vi "RegisterWindow.vi"() -> ()   [LabVIEW 2013]
panel:
  out "子字符串":string
  out "LicCode":string
  out "机器码":string
  out "Tip":string
  in  "注册码":string
  out "连接的字符串":string
  in  "退出":bool
  in  "注册":bool
  in  "簇":T1
  out "字符串":string
  out "鉴权通过":bool
  out "参数配置":bool
  out "参数生成":bool
  out "强制操作":bool
  out "数据保存":bool
  out "Times":dbl
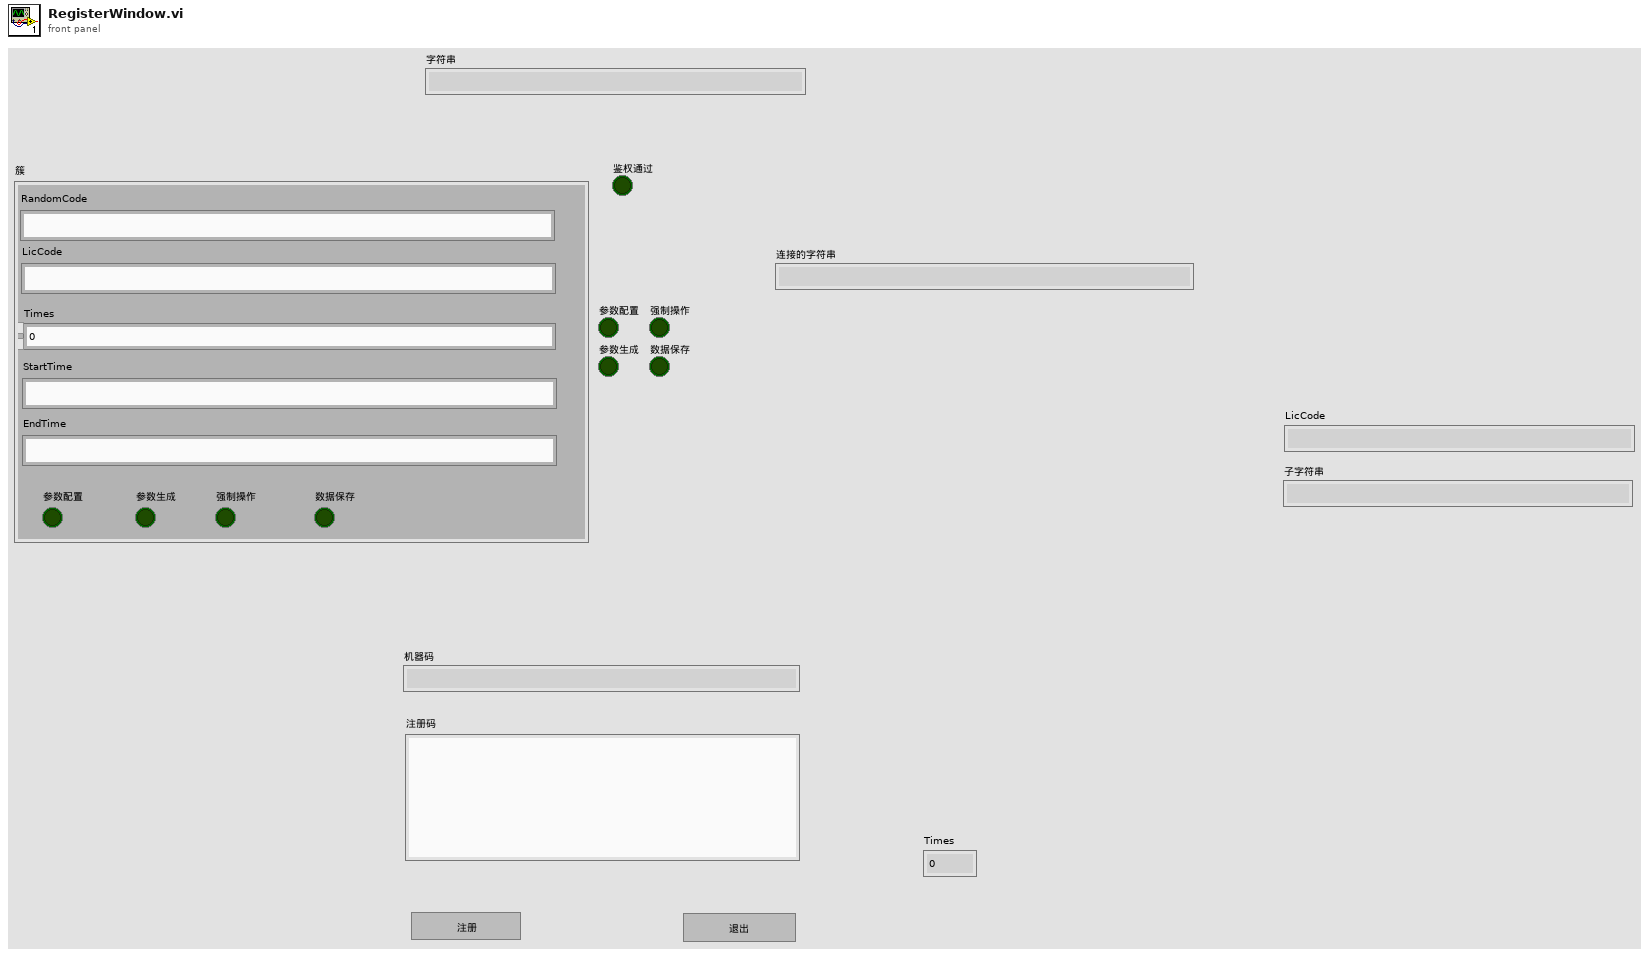
[diagram p1: front panel]
types:
  T1 = cluster{"RandomCode":string, "LicCode":string, "Times":dbl, "StartTime":string, "EndTime":string, "参数配置":bool, "参数生成":bool, "强制操作":bool, "数据保存":bool}
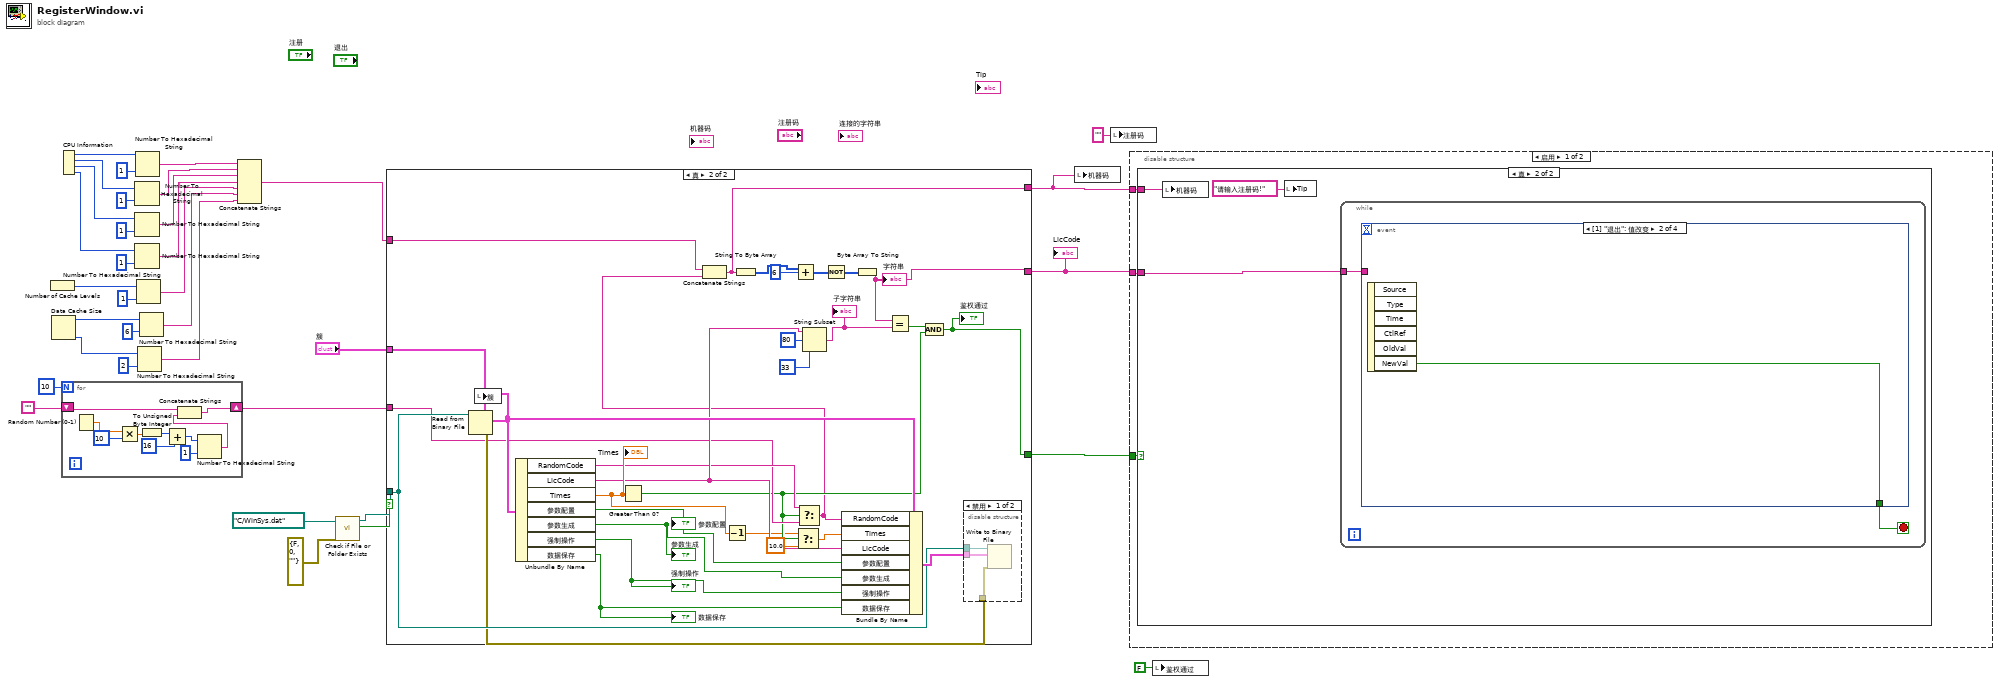
[diagram p0: block diagram]
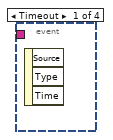
[diagram p3: hidden frame]
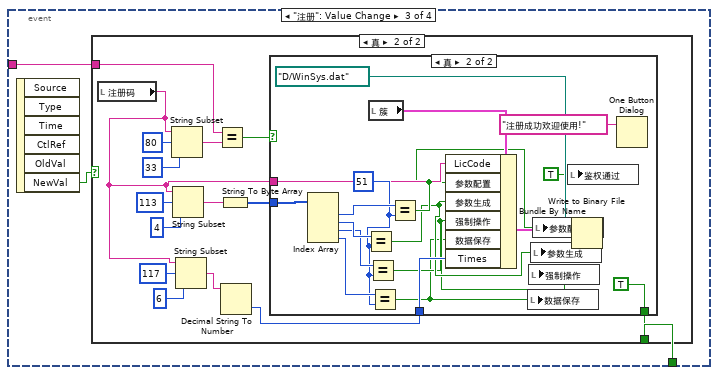
[diagram p4: hidden frame]
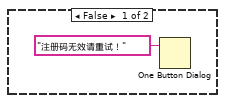
[diagram p6: hidden frame]
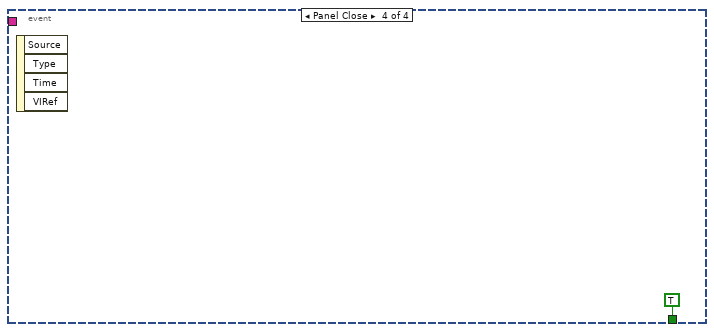
[diagram p7: hidden frame]
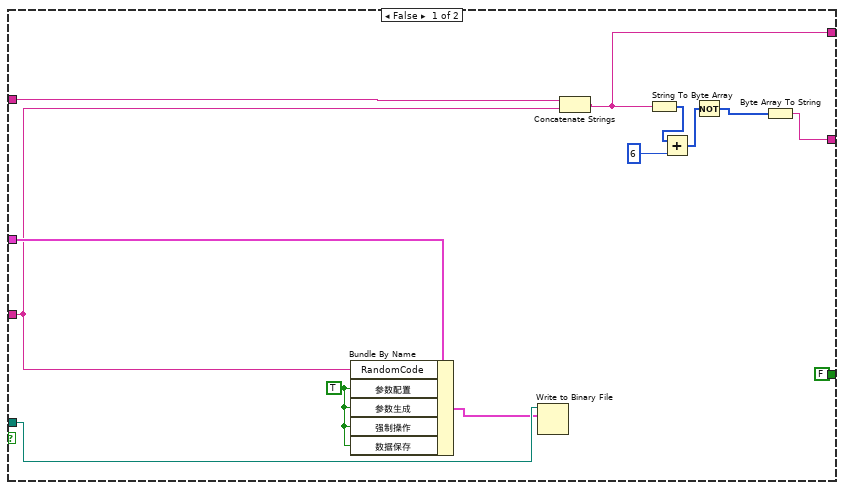
[diagram p9: hidden frame]
diagram:
  n1 = Number of Cache Levels() -> (w20:i32)
  n2 = Data Cache Size() -> (4:w21:i32, 7:w23:i32)  [unwired: 1 in]
  n3 = CPU Information() -> (4:w11:i32, 5:w15:i32, 6:w16:i32, 7:w17:i32)
  n4 = for {
    N: 10 -> [_]
    shift-right: [w37] -> w1
    shift-left: "" -> [w38]
    n5 = Random Number (0-1)() -> (number: 0 to 1=w45:dbl)
    n6 = Multiply(x=w45, y=u8 10) -> (x*y=w43:dbl)
    n7 = To Unsigned Byte Integer(number=w43) -> (unsigned 8bit integer=w41:u8)
    n8 = Add(x=w41, y=u8 16) -> (x+y=w39:u8)
    n9 = Number To Hexadecimal String(1:i16 1 ("宽度(-)"), 2:w39) -> (0:w36:string)
    n10 = Concatenate Strings(w38, w36) -> (w37:string)
  }
  n11 = Number To Hexadecimal String(1:i16 1 ("宽度(-)"), 2:w15) -> (0:w25:string)
  n12 = Number To Hexadecimal String(1:i16 1 ("宽度(-)"), 2:w16) -> (0:w26:string)
  n13 = Number To Hexadecimal String(1:i16 1 ("宽度(-)"), 2:w17) -> (0:w27:string)
  n14 = Number To Hexadecimal String(1:i16 1 ("宽度(-)"), 2:w11) -> (0:w24:string)
  n15 = Number To Hexadecimal String(1:i16 1 ("宽度(-)"), 2:w20) -> (0:w28:string)
  n16 = Number To Hexadecimal String(1:i16 2 ("宽度(-)"), 2:w23) -> (0:w30:string)
  n17 = Number To Hexadecimal String(1:i16 6 ("宽度(-)"), 2:w21) -> (0:w29:string)
  n18 = Concatenate Strings(w24, w25, w26, w27, w28, w29, w30) -> (w9:string)
  n19 = call <vilib>:"Check if File or Folder Exists.vi"("error in (no error)"=errorcluster {"status"=FALSE, "code"=0, "source"=""}, "path"=path "C:/WinSys.dat" ("文件（使用对话框）")) -> ("file or folder exists?"=w33:bool, "dup path"=w32:path)  [unwired: 7 in, 1 out]
  n20 = case shown="真" w33 {
    tunnel: w32 -> [w57 w73]
    tunnel: "簇" -> [w55 w86]
    tunnel: w9 -> [w52 w83]
    tunnel: [FALSE w77] -> w8
    tunnel: [w48 w76] -> w7
    tunnel: [w47 w75] -> w5
    tunnel: w1 -> [w46 w63]
    frame False {
      w54 = TRUE ("参数配置")
      n21 = Bundle By Name(cluster=w55, "RandomCode"=w46, "参数配置"=w54, "参数生成"=w54, "强制操作"=w54, "数据保存"=w54) -> (w56:T1)
      n22 = Write to Binary File(file (use dialog)=w57, data=w56) -> ()  [unwired: 4 in, 3 out]
      n23 = Concatenate Strings(w52, w46) -> (w47:string)
      n24 = String To Byte Array(string=w47) -> (unsigned byte array=w51:u8[])
      n25 = Add(x=w51, y=u8 6) -> (x+y=w49:u8[])
      n26 = Not(x=w49) -> ()  [unwired: 1 out]
      n27 = Byte Array To String(unsigned byte array=w49) -> (string=w48:string)
    }
    frame True {
      n28 = Read from Binary File(5:w86, 11:w73) -> (0:w65:errorcluster, 2:w72:T1)  [unwired: 4 in, 2 out]
      n29 = local write "簇"(w72) -> ()
      n30 = Unbundle By Name(w72) -> ("RandomCode"=w64:string, "LicCode"=w66:string, "Times"=w71:dbl, "参数配置"=w70:bool, "参数生成"=w69:bool, "强制操作"=w68:bool, "数据保存"=w67:bool)
      "参数配置" <- w70
      "参数生成" <- w69
      "强制操作" <- w68
      "数据保存" <- w67
      "Times" <- w71
      n31 = Greater Than 0?(x=w71) -> (x > 0?=w62:bool)
      n32 = Decrement(x=w71) -> (x-1=w60:dbl)
      n33 = Select(t=w60, s=w62, f=10.0) -> (s? t:f=w61:dbl)
      n34 = Select(t=w64, s=w62, f=w63) -> (s? t:f=w58:string)
      n35 = Concatenate Strings(w83, w58) -> (w75:string)
      n36 = String To Byte Array(string=w75) -> (unsigned byte array=w82:u8[])
      n37 = Add(x=w82, y=u8 6) -> (x+y=w80:u8[])
      n38 = String Subset(string=w66, offset (0)=80 ("偏移量(0)"), length (rest)=33 ("长度（剩余）")) -> (substring=w79:string)
      "子字符串" <- w79
      n39 = Not(x=w80) -> ()  [unwired: 1 out]
      n40 = Bundle By Name(cluster=w72, "RandomCode"=w58, "Times"=w61, "LicCode"=w66, "参数配置"=w70, "参数生成"=w69, "强制操作"=w68, "数据保存"=w67) -> (w74:T1)
      n41 = Byte Array To String(unsigned byte array=w80) -> (string=w76:string)
      "字符串" <- w76
      n42 = Equal?(x=w76, y=w79) -> (x = y?=w78:bool)
      n43 = And(x=w78, y=w62) -> (x .and. y?=w77:bool)
      "鉴权通过" <- w77
      n44 = disable-structure shown="禁用" {
        disable-tunnel: w74 -> [w89 _]
        disable-tunnel: w73 -> [w88 _]
        disable-tunnel: w65 -> [w87 _]
        frame Disabled {
          n45 = Write to Binary File(file (use dialog)=w88, data=w89, error in=w87) -> ()  [unwired: 3 in, 3 out]
        }
        frame Enabled {
        }
      }
    }
  }
  "LicCode" <- w7
  n46 = local write "机器码"(w5) -> ()
  n47 = local write "注册码"("" ("注册码")) -> ()
  n48 = disable-structure shown="启用" {
    disable-tunnel: w8 -> [w92 _]
    disable-tunnel: w7 -> [w91 _]
    disable-tunnel: w5 -> [w90 _]
    frame Enabled {
      n49 = case shown="真" w92 {
        tunnel: w91 -> [_ w95]
        tunnel: w90 -> [_ w93]
        frame False {
        }
        frame True {
          n50 = local write "机器码"(w93) -> ()
          n51 = local write "Tip"("请输入注册码!" ("Tip")) -> ()
          n52 = while {
            tunnel: w95 -> [w97]
            stop <- w96 stop-if-true
            n53 = event shown="[1] \"退出\": 值改变" {
              selector: _ -> [_ _ _ _]
              dyn-events: _ -> [_ _ _ _]
              timeout: _ -> [_ _ _ _]
              tunnel: w97 -> [_ _ w101 _]
              tunnel: [_ w98 w100 TRUE ("新值")] -> w96
              event Timeout {
                n54 = event-data() -> ()  [unwired: 1 in, 3 out]
              }
              event "退出": Value Change {
                n55 = event-data() -> ("NewVal"=w98:bool)  [unwired: 1 in, 5 out]
              }
              event "注册": Value Change {
                n56 = event-data() -> ("NewVal"=w99:bool)  [unwired: 1 in, 5 out]
                n57 = case shown="真" w99 {
                  tunnel: w101 -> [_ w113]
                  tunnel: [_ w102] -> w100
                  frame False {
                  }
                  frame True {
                    n58 = local read "注册码"() -> (w105:string)
                    n59 = String Subset(string=w105, offset (0)=80 ("偏移量(0)"), length (rest)=33 ("长度（剩余）")) -> (substring=w116:string)
                    n60 = String Subset(string=w105, offset (0)=113 ("偏移量(0)"), length (rest)=4 ("长度（剩余）")) -> (substring=w109:string)
                    n61 = String Subset(string=w105, offset (0)=117 ("偏移量(0)"), length (rest)=6 ("长度（剩余）")) -> (substring=w104:string)
                    n62 = Equal?(x=w113, y=w116) -> (x = y?=w112:bool)
                    n63 = String To Byte Array(string=w109) -> (unsigned byte array=w108:u8[])
                    n64 = Decimal String To Number(string=w104) -> (number=w103:i32)  [unwired: 2 in, 1 out]
                    n65 = case shown="真" w112 {
                      tunnel: w108 -> [_ w132]
                      tunnel: w105 -> [_ w126]
                      tunnel: w103 -> [_ w125]
                      tunnel: [_ TRUE ("新值")] -> w102
                      frame False {
                        n66 = One Button Dialog(message="注册码无效请重试！" ("消息")) -> ()  [unwired: 1 in, 1 out]
                      }
                      frame True {
                        w127 = 51 ("索引")
                        n67 = Index Array(array=w132) -> (element #1=w131:u8, element #2=w130:u8, element #3=w129:u8, element #4=w128:u8)  [unwired: 4 in]
                        n68 = Equal?(x=w130, y=w127) -> (x = y?=w120:bool)
                        n69 = Equal?(x=w129, y=w127) -> (x = y?=w119:bool)
                        n70 = local read "簇"() -> (w133:T1)
                        n71 = Equal?(x=w128, y=w127) -> (x = y?=w118:bool)
                        n72 = Equal?(x=w131, y=w127) -> (x = y?=w121:bool)
                        n73 = Bundle By Name(cluster=w133, "LicCode"=w126, "参数配置"=w121, "参数生成"=w120, "强制操作"=w119, "数据保存"=w118, "Times"=w125) -> (w135:T1)
                        n74 = local write "数据保存"(w118) -> ()
                        n75 = local write "强制操作"(w119) -> ()
                        n76 = local write "参数生成"(w120) -> ()
                        n77 = local write "参数配置"(w121) -> ()
                        n78 = local write "鉴权通过"(TRUE ("鉴权通过")) -> ()
                        n79 = Write to Binary File(file (use dialog)=path "D:/WinSys.dat" ("文件（使用对话框）"), data=w135) -> ()  [unwired: 4 in, 3 out]
                        n80 = One Button Dialog(message="注册成功欢迎使用!" ("消息")) -> ()  [unwired: 1 in, 1 out]
                      }
                    }
                  }
                }
              }
              event Panel Close {
                n81 = event-data() -> ()  [unwired: 1 in, 4 out]
              }
            }
          }
        }
      }
    }
    frame Disabled {
    }
  }
  n82 = local write "鉴权通过"(FALSE ("鉴权通过")) -> ()
